vi "Version 1_Read Measurements.vi"(7 "Address (A)":string="A", 8 "error in":errorcluster, 9 "Totalizer Timer":enum32{"Disable", "Enable"}(radio)=enum."Enable", 10 "Data Flags In":T2, 11 "VISA Session In":refnum<visa-resource-name>="Alicat") -> (0 "error out":errorcluster, 1 "Data":T1={"Identifier"="", "Pressure"=nan, "Temperature"=nan, "Volumetric"=nan, "Mass"=nan, "SetPoint"=nan, "Valve Drive"=nan, "Totalizer"=nan, "Gas"="", "Totalizer Timer"=""} {"Valve Drive" format="%#_6f"; "Totalizer" format="%#_6f"; "SetPoint" format="%#_6f"; "Pressure" format="%#_6f"; "Temperature" format="%#_6f"; "Volumetric" format="%#_6f"; "Mass" format="%#_6f"}, 2 "Data Flags Out":T2, 3 "VISA Session Out":refnum<visa-resource-name>, 4 "Overrange":T4, 6 "Faults/Status":T3)   [LabVIEW 2016]
uses:
  Measurements.ctl
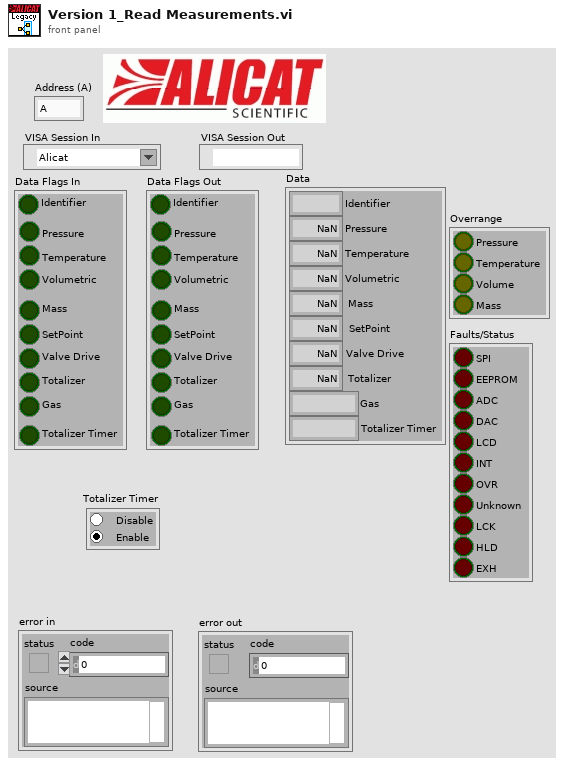
[diagram p1: front panel]
types:
  T1 = typedef "Measurements.ctl" = cluster{"Identifier":string, "Pressure":dbl, "Temperature":dbl, "Volumetric":dbl, "Mass":dbl, "SetPoint":dbl, "Valve Drive":dbl, "Totalizer":dbl, "Gas":string, "Totalizer Timer":string}
  T2 = cluster{"Identifier":bool, "Pressure":bool, "Temperature":bool, "Volumetric":bool, "Mass":bool, "SetPoint":bool, "Valve Drive":bool, "Totalizer":bool, "Gas":bool, "Totalizer Timer":bool}
  T3 = cluster{"SPI":bool, "EEPROM":bool, "ADC":bool, "DAC":bool, "LCD":bool, "INT":bool, "OVR":bool, "Unknown":bool, "LCK":bool, "HLD":bool, "EXH":bool}
  T4 = cluster{"Pressure":bool, "Temperature":bool, "Volume":bool, "Mass":bool}
  T5 = cluster{"Absolute Pressure":bool, "Gauge/Diff. Pressure":bool, "Barometric Pressure":bool, "Temperature":bool, "Volumetric":bool, "Mass":bool, "Setpoint":bool, "Valve Drive":bool, "Totalizer":bool, "Totalizer Timer":bool, "Totalizer Average Flow":bool, "Totalizer Peak Flow":bool, "Gas Selected":bool, "Tot. Timer Format":u16}
  T6 = typedef "Data Frame.ctl" = cluster{"Absolute Pressure":bool, "Gauge/Diff. Pressure":bool, "Barometric Pressure":bool, "Temperature":bool, "Volumetric":bool, "Mass":bool, "Setpoint":bool, "Valve Drive":bool, "Totalizer":bool, "Totalizer Timer":bool, "Totalizer Average Flow":bool, "Totalizer Peak Flow":bool, "Gas Selected":bool, "Tot. Timer Format":u16}
  T7 = typedef "Data Cluster.ctl" = cluster{"Absolute Pressure":dbl, "Gauge/Diff. Pressure":dbl, "Barometric Pressure":dbl, "Temperature":dbl, "Volumetric Flow":dbl, "Mass Flow":dbl, "Setpoint":dbl, "Valve Drive":dbl, "Totalizer":dbl, "[hr]":dbl, "[min]":dbl, "[sec]":dbl, "Totalizer Average Flow":dbl, "Totalizer Peak Flow":dbl, "Gas selected":string}
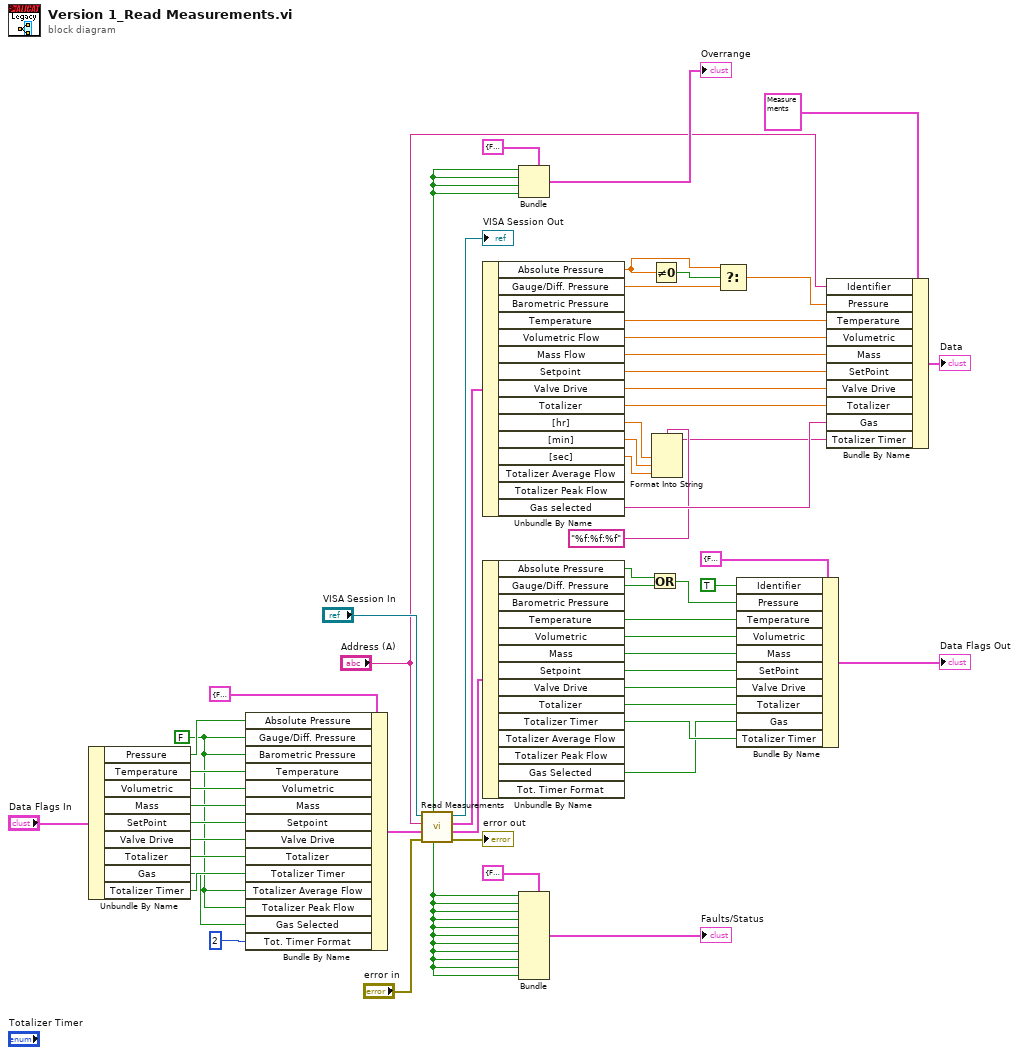
[diagram p0: block diagram]
diagram:
  w42 = FALSE ("Totalizer Peak Flow")
  n1 = Unbundle By Name("Data Flags In") -> ("Pressure"=w43:bool, "Temperature"=w44:bool, "Volumetric"=w45:bool, "Mass"=w46:bool, "SetPoint"=w47:bool, "Valve Drive"=w48:bool, "Totalizer"=w50:bool, "Gas"=w49:bool, "Totalizer Timer"=w51:bool)
  n2 = Bundle By Name(cluster=T5 {"Absolute Pressure"=FALSE, "Gauge/Diff. Pressure"=FALSE, "Barometric Pressure"=FALSE, "Temperature"=FALSE, "Volumetric"=FALSE, "Mass"=FALSE, "Setpoint"=FALSE, "Valve Drive"=FALSE, "Totalizer"=FALSE, "Totalizer Timer"=FALSE, "Totalizer Average Flow"=FALSE, "Totalizer Peak Flow"=FALSE, "Gas Selected"=FALSE, "Tot. Timer Format"=0} ("Data Frame Format In"), "Absolute Pressure"=w43, "Gauge/Diff. Pressure"=w42, "Barometric Pressure"=w42, "Temperature"=w44, "Volumetric"=w45, "Mass"=w46, "Setpoint"=w47, "Valve Drive"=w48, "Totalizer"=w50, "Totalizer Timer"=w51, "Totalizer Average Flow"=w42, "Totalizer Peak Flow"=w42, "Gas Selected"=w49, "Tot. Timer Format"=u16 2) -> (w18:T5)
  n3 = call "Read Measurements.vi"("error in"="error in", "Data Frame Format In"=w18, "Unit ID (A)"="Address (A)", "VISA Session In"="VISA Session In") -> ("error out"=→"error out":errorcluster, "Data Frame Format Out"=w55:T6, "Data Cluster"=w19:T7, "VISA Session Out"=→"VISA Session Out":refnum<visa-resource-name>, "Error Present"=w22:bool, "Range Exceeded"=w25:bool)  [unwired: 2 out]
  n4 = Unbundle By Name(w19) -> ("Absolute Pressure"=w10:dbl, "Gauge/Diff. Pressure"=w9:dbl, "Temperature"=w7:dbl, "Volumetric Flow"=w6:dbl, "Mass Flow"=w5:dbl, "Setpoint"=w4:dbl, "Valve Drive"=w3:dbl, "Totalizer"=w2:dbl, "[hr]"=w15:dbl, "[min]"=w14:dbl, "[sec]"=w13:dbl, "Gas selected"=w17:string)  [unwired: 3 out]
  n5 = Unbundle By Name(w55) -> ("Absolute Pressure"=w31:bool, "Gauge/Diff. Pressure"=w30:bool, "Temperature"=w33:bool, "Volumetric"=w34:bool, "Mass"=w35:bool, "Setpoint"=w36:bool, "Valve Drive"=w37:bool, "Totalizer"=w39:bool, "Totalizer Timer"=w40:bool, "Gas Selected"=w38:bool)  [unwired: 4 out]
  n6 = Bundle(cluster=T4 {"Pressure"=FALSE, "Temperature"=FALSE, "Volume"=FALSE, "Mass"=FALSE} ("Overrange"), "Pressure"=w25, "Temperature"=w25, "Volume"=w25, "Mass"=w25) -> (→"Overrange":T4)
  n7 = Bundle(cluster=T3 {"SPI"=FALSE, "EEPROM"=FALSE, "ADC"=FALSE, "DAC"=FALSE, "LCD"=FALSE, "INT"=FALSE, "OVR"=FALSE, "Unknown"=FALSE, "LCK"=FALSE, "HLD"=FALSE, "EXH"=FALSE} ("Faults/Status"), "SPI"=w22, "EEPROM"=w22, "ADC"=w22, "DAC"=w22, "LCD"=w22, "INT"=w22, "OVR"=w22, "Unknown"=w22, "LCK"=w22, "HLD"=w22, "EXH"=w22) -> (→"Faults/Status":T3)
  n8 = Or(x=w31, y=w30) -> (x .or. y?=w29:bool)
  n9 = Not Equal To 0?(x=w10) -> (x != 0?=w11:bool)
  n10 = Format Into String(format string="%f:%f:%f", w15, w14, w13) -> (resulting string=w12:string)  [unwired: 2 in, 1 out]
  n11 = Select(t=w10, s=w11, f=w9) -> (s? t:f=w8:dbl)
  n12 = Bundle By Name(cluster=T2 {"Identifier"=FALSE, "Pressure"=FALSE, "Temperature"=FALSE, "Volumetric"=FALSE, "Mass"=FALSE, "SetPoint"=FALSE, "Valve Drive"=FALSE, "Totalizer"=FALSE, "Gas"=FALSE, "Totalizer Timer"=FALSE} ("Data Flags Out"), "Identifier"=TRUE, "Pressure"=w29, "Temperature"=w33, "Volumetric"=w34, "Mass"=w35, "SetPoint"=w36, "Valve Drive"=w37, "Totalizer"=w39, "Gas"=w38, "Totalizer Timer"=w40) -> (→"Data Flags Out":T2)
  n13 = Bundle By Name(cluster=T1 {"Identifier"="", "Pressure"=nan, "Temperature"=nan, "Volumetric"=nan, "Mass"=nan, "SetPoint"=nan, "Valve Drive"=nan, "Totalizer"=nan, "Gas"="", "Totalizer Timer"=""} ("Data"), "Identifier"="Address (A)", "Pressure"=w8, "Temperature"=w7, "Volumetric"=w6, "Mass"=w5, "SetPoint"=w4, "Valve Drive"=w3, "Totalizer"=w2, "Gas"=w17, "Totalizer Timer"=w12) -> (→"Data":T1)
